vi "myRIO v1.0 Close UART.vi"(8 "error in (no error)":errorcluster, 11 "VISA resource array":refnum<visa-resource-name>[](array[refnum])) -> (0 "error out":errorcluster)   [LabVIEW 2021]
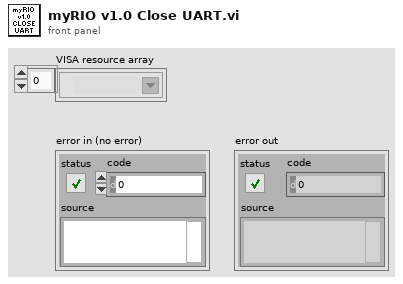
[diagram p1: front panel]
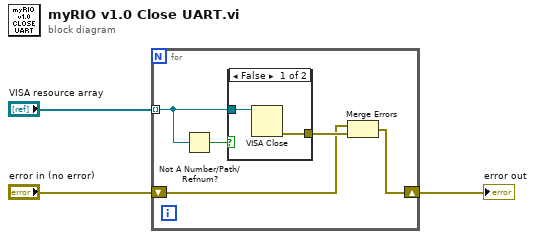
[diagram p0: block diagram]
diagram:
  n1 = for {
    tunnel: "VISA resource array" -> [w7] mode=indexing
    shift-right: [w4] -> w2
    shift-left: "error in (no error)" -> [w5]
    n2 = Not A Number/Path/Refnum?(number/path/refnum=w7) -> (NaN/Path/Refnum?=w8:bool)
    n3 = case shown="False" w8 {
      tunnel: w7 -> [w10 _]
      tunnel: [w9 _] -> w6
      frame False {
        n4 = VISA Close(VISA resource name=w10) -> (error out=w9:errorcluster)  [unwired: 1 in]
      }
      frame True {
      }
    }
    n5 = Merge Errors(w5, w6) -> (w4:errorcluster)
  }
  "error out" <- w2
